vi "Load Configuration Information for UI.vi"(8 "error in (no error)":errorcluster, 11 "node in":refnum<class "RIO Target.lvclass">) -> (0 "error out":errorcluster, 2 "UI Configuration":T1, 3 "node out":refnum<class "RIO Target.lvclass">)   [LabVIEW 2014, in "RIO Target.lvclass"]
uses:
  RIO Target.lvclass
  UI Configuration.ctl
  RIO Target.lvclass/RIO Target.ctl
  RIO Target Configuration/RIO Target Configuration.lvclass/RIO Target Configuration.ctl
  RIO Target Configuration/RIO Target Configuration.lvclass
  <vilib>/NI/Configuration Framework/serializable configuration/NISE_CEF_serializable configuration.lvclass
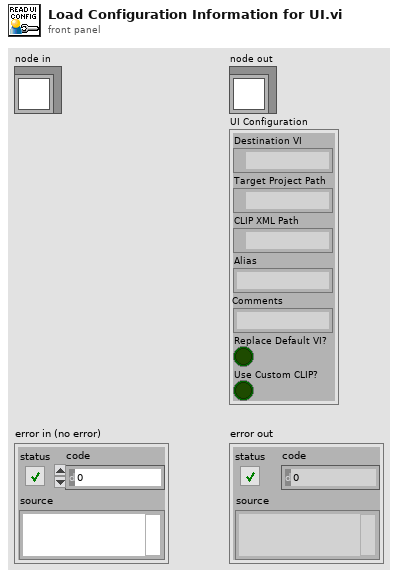
[diagram p1: front panel]
types:
  T1 = typedef "RIO Target.lvclass/UI Configuration.ctl" = cluster{"Destination VI":path, "Target Project Path":path, "CLIP XML Path":path, "Alias":string, "Comments":string, "Replace Default VI?":bool, "Use Custom CLIP?":bool}
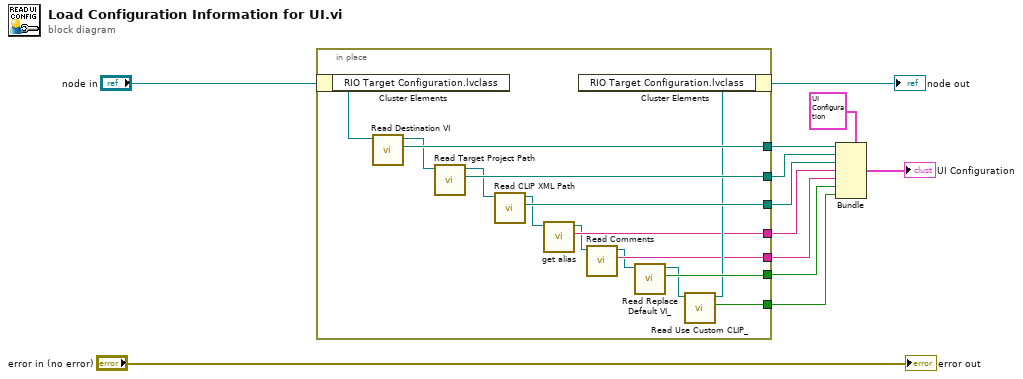
[diagram p0: block diagram]
diagram:
  n1 = in-place {
    in-place-border: [w26] -> w11
    in-place-border: [w24] -> w10
    in-place-border: [w22] -> w9
    in-place-border: [w17] -> w8
    in-place-border: [w21] -> w2
    in-place-border: [w19] -> w1
    in-place-border: [w15] -> w3
    n2 = in-place-cluster #1("node in") -> ("RIO Target Configuration.lvclass"=w27:refnum<class "RIO Target Configuration.lvclass">)
    n3 = call "Read Destination VI.vi"("RIO Target Configuration in"=w27) -> ("Destination VI"=w26:path, "RIO Target Configuration out"=w25:refnum<class "RIO Target Configuration.lvclass">)  [unwired: 8 in, 1 out]
    n4 = call "Read Target Project Path.vi"("RIO Target Configuration in"=w25) -> ("Target Project Path"=w24:path, "RIO Target Configuration out"=w23:refnum<class "RIO Target Configuration.lvclass">)  [unwired: 8 in, 1 out]
    n5 = call "Read CLIP XML Path.vi"("RIO Target Configuration in"=w23) -> ("CLIP XML Path"=w22:path, "RIO Target Configuration out"=w16:refnum<class "RIO Target Configuration.lvclass">)  [unwired: 8 in, 1 out]
    n6 = call <vilib>:"get alias.vi"("configuration in"=w16) -> ("alias"=w17:string, "configuration out"=w14:refnum<class "RIO Target Configuration.lvclass">)  [unwired: 8 in, 1 out]
    n7 = call "Read Comments.vi"("RIO Target Configuration in"=w14) -> ("Comments"=w15:string, "RIO Target Configuration out"=w13:refnum<class "RIO Target Configuration.lvclass">)  [unwired: 8 in, 1 out]
    n8 = call "Read Replace Default VI_.vi"("RIO Target Configuration in"=w13) -> ("Replace Default VI?"=w21:bool, "RIO Target Configuration out"=w20:refnum<class "RIO Target Configuration.lvclass">)  [unwired: 8 in, 1 out]
    n9 = call "Read Use Custom CLIP_.vi"("RIO Target Configuration in"=w20) -> ("Use Custom CLIP?"=w19:bool, "RIO Target Configuration out"=w18:refnum<class "RIO Target Configuration.lvclass">)  [unwired: 8 in, 1 out]
    n10 = in-place-cluster #1("RIO Target Configuration.lvclass"=w18) -> (→"node out":refnum<class "RIO Target.lvclass">)
  }
  n11 = Bundle(cluster=T1 {"Destination VI"=path "", "Target Project Path"=path "", "CLIP XML Path"=path "", "Alias"="", "Comments"="", "Replace Default VI?"=FALSE, "Use Custom CLIP?"=FALSE} ("output cluster"), "Destination VI"=w11, "Target Project Path"=w10, "CLIP XML Path"=w9, "Alias"=w8, "Comments"=w3, "Replace Default VI?"=w2, "Use Custom CLIP?"=w1) -> (→"UI Configuration":T1)
  "error out" <- "error in (no error)"
